vi "TSM DMM Close Sessions.vi"(0 "TSM context":T1) -> (15 "error out":errorcluster)   [LabVIEW 2020]
doc: "Use this VI to reset and close all sessions for all NI-DMM instruments in the Semiconductor Module Context."
uses:
  <vilib>/NI_TestStand_SemiconductorModule/NI_TestStand_Semiconductor_Module.lvlibp/PinMap/General/SemiconductorModuleContext.ctl
  <vilib>/NI_TestStand_SemiconductorModule/NI_TestStand_Semiconductor_Module.lvlibp
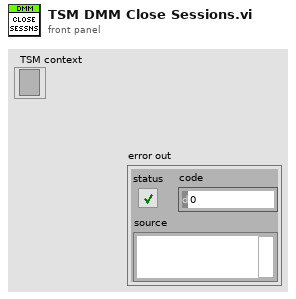
[diagram p1: front panel]
types:
  T1 = typedef "NI_TestStand_Semiconductor_Module.lvlibp/SemiconductorModuleContext.ctl" = refnum<k7>
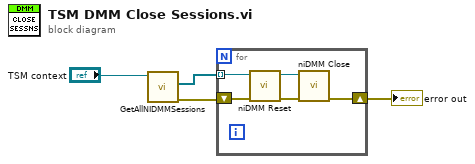
[diagram p0: block diagram]
diagram:
  n1 = call <vilib>:"GetAllNIDMMSessions.vi"("Semiconductor Module Context"="TSM context") -> ("error out"=w4:errorcluster, "Instrument Sessions"=w3:refnum<k15>[])  [unwired: 8 in, 1 out]
  n2 = for {
    tunnel: w3 -> [w6] mode=indexing
    shift-right: [w8] -> w1
    shift-left: w4 -> [w9]
    n3 = call <instrlib>:"niDMM Reset.vi"("error in (no error)"=w9, "instrument handle"=w6) -> ("error out"=w7:errorcluster, "instrument handle out"=w5:refnum<k15>)  [unwired: 8 in]
    n4 = call <instrlib>:"niDMM Close.vi"("error in (no error)"=w7, "instrument handle"=w5) -> ("error out"=w8:errorcluster)  [unwired: 9 in]
  }
  "error out" <- w1
